vi "Get Default Value.vi"(6 "Data Type":T1, 8 "error in (no error)":errorcluster, 11 "Floating Point in":refnum<class "Floating Point.lvclass">) -> (0 "error out":errorcluster, 2 "Data Value":variant)   [LabVIEW 2018, in "Floating Point.lvclass"]
doc: "Gets a default value for each data type and passes it out to be set by Add Test Parameter"
uses:
  Floating Point.lvclass
  <vilib>/Utility/Data Type/Type Definitions/Data Type.ctl
  <vilib>/Utility/Data Type/NI_Data Type.lvlib
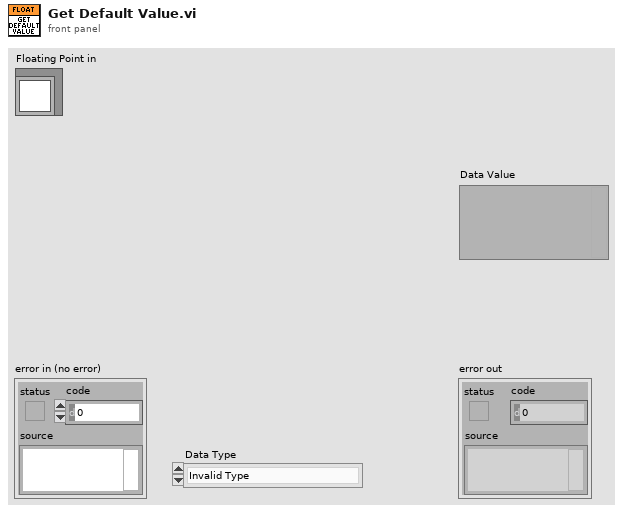
[diagram p1: front panel]
types:
  T1 = typedef "NI_Data Type.lvlib/Data Type.ctl" = enum8{"Invalid Type", "Void", "I8", "I16", "I32", "I64", "U8", "U16", "U32", "U64", "Single Float", "Double Float", "Extended Float", "Single Complex", "Double Complex", "Extended Complex", "Enum U8", "Enum U16", "Enum U32", "Enum U64", "Single Float With Unit", "Double Float With Unit", "Extended Float With Unit", "Single Complex with Unit", "Double Complex with Unit", "Extended Complex with Unit", "Boolean", "String", "Path", "Picture", "Tag", "Array", "Cluster", "Variant", "LV Variant", "Waveform", "Timestamp", "Digital Waveform", "Digital Data", "ExpressData", "Refnum", "External Data", "VI", "Poly VI", "LabVIEW Class Instance", "Fixed Point"}
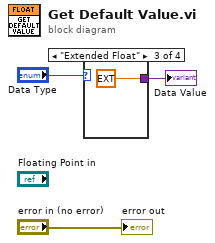
[diagram p0: block diagram]
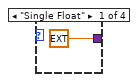
[diagram p2: hidden frame]
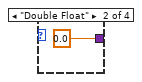
[diagram p3: hidden frame]
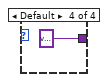
[diagram p4: hidden frame]
diagram:
  n1 = case shown="\"Extended Float\"" "Data Type" {
    tunnel: [ext 0.0 0.0 ext 0.0 variant] -> w1
    frame "Single Float" {
    }
    frame "Double Float" {
    }
    frame "Extended Float" {
    }
    frame Default {
    }
  }
  "Data Value" <- w1
  "error out" <- "error in (no error)"
